vi "Send Parameter Message.vi"(5 "Write?":bool, 7 "Param Address":i16, 9 "Data":u16, 10 "CAN Offset":u32=160 format="%x", 11 "CANTXQueueIn":T1) -> (3 "CANTXQueueOut":T1)   [LabVIEW 2015]
uses:
  TX Library/CAN Message Queue.ctl
  TX Library/CAN Message.ctl
  <vilib>/RioEmbeddedCAN/RioEmbeddedCAN.llb/CANFrameControl.ctl
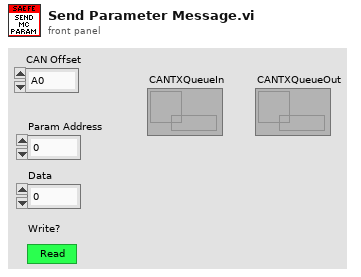
[diagram p1: front panel]
types:
  T1 = typedef "CAN Message Queue.ctl" = refnum<k33>
  T2 = typedef "CANFrameControl.ctl" = cluster{"identifier":u32, "extended?":bool, "type":u8, "payload":u8[]}
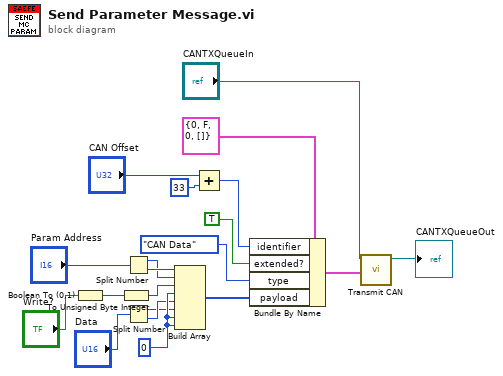
[diagram p0: block diagram]
diagram:
  w16 = u8 0 ("element")
  n1 = Boolean To (0,1)(Boolean="Write?") -> (0, 1=w17:i16)
  n2 = To Unsigned Byte Integer(number=w17) -> (unsigned 8bit integer=w18:u8)
  n3 = Split Number(x="Param Address") -> (hi(x)=w4:u8, lo(x)=w5:u8)
  n4 = Split Number(x="Data") -> (hi(x)=w13:u8, lo(x)=w14:u8)
  n5 = Build Array(w5, w4, w18, w16, w14, w13, w16, w16) -> (w11:u8[])
  n6 = Add(x="CAN Offset", y=u32 33) -> (x+y=w6:u32)
  n7 = Bundle By Name(cluster=T2 {"identifier"=0, "extended?"=FALSE, "type"=0, "payload"=[]} ("CAN frame"), "identifier"=w6, "extended?"=TRUE, "type"=enum8{"CAN Data", "CAN Remote"}."CAN Data", "payload"=w11) -> (w3:T2)
  n8 = call "Transmit CAN.vi"("CAN Queue"="CANTXQueueIn", "CAN frame"=w3) -> ("CAN Queue Out"=→"CANTXQueueOut":T1)  [unwired: 8 in]
